vi "InitializePathsByIndex.vi"(8 "error in (no error)":errorcluster, 10 "Paths":string[](array[string]), 11 "Setting Database in":refnum<class "Setting Database.lvclass">) -> (0 "error out":errorcluster, 3 "Setting Database out":refnum<class "Setting Database.lvclass">)   [LabVIEW 2019, in "Setting Database.lvclass"]
uses:
  Setting Database.lvclass
  Setting Database.lvclass/Setting Database.ctl
  Path Settings/Path Settings.lvclass
  C:/Users/Albro/Documents/GitHub/AFM-Lithography/lvsrc/Classes/Settings/ObjectSettings/ObjectSettings.lvclass
  <vilib>/Utility/sysdir.llb/Get System Directory.vi
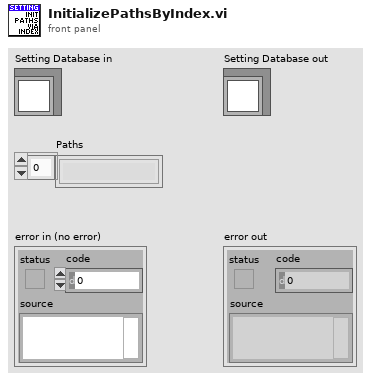
[diagram p1: front panel]
types:
  T1 = cluster{"Path":i32, "Funnel":i32, "Rectangle":i32, "Dot":i32}
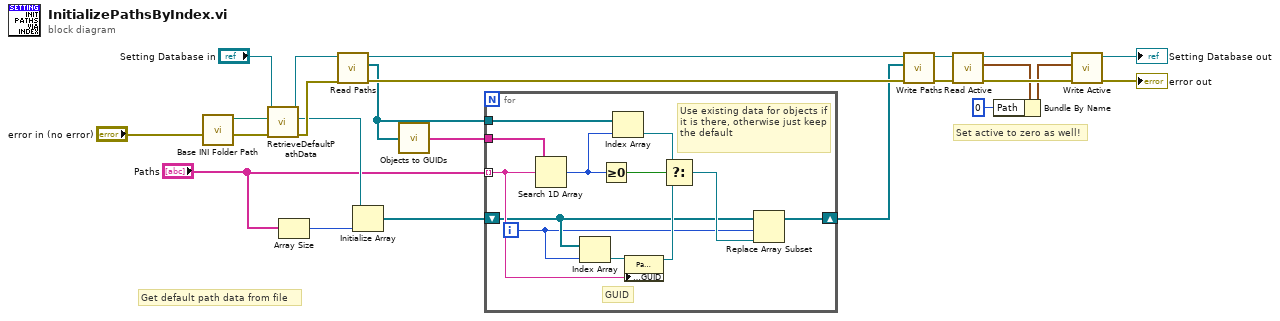
[diagram p0: block diagram]
diagram:
  # "Get default path data from file"
  # "Set active to zero as well!"
  n1 = call "Base INI Folder Path.vi"() -> ("Base Path"=w7:path)  [unwired: 11 in]
  n2 = call "RetrieveDefaultPathData.vi"("error in (no error)"="error in (no error)", "Path"=w7, "Setting Database In"="Setting Database in") -> ("error out"=w11:errorcluster, "Path Settings"=w8:refnum<class "Path Settings.lvclass">, "Setting Database Out"=w9:refnum<class "Setting Database.lvclass">)  [unwired: 6 in]
  n3 = Array Size(array="Paths") -> (size(s)=w6:i32)
  n4 = call "Read Paths.vi"("error in (no error)"=w11, "Setting Database in"=w9) -> ("error out"=w21:errorcluster, "Paths"=w5:refnum<class "Path Settings.lvclass">[], "Setting Database out"=w22:refnum<class "Setting Database.lvclass">)  [unwired: 7 in]
  n5 = Initialize Array(w8, w6) -> (w2:refnum<class "Path Settings.lvclass">[])
  n6 = call "Objects to GUIDs.vi"("Objects"=w5) -> ("GUIDs"=w4:string[])  [unwired: 3 in, 1 out]
  n7 = for {
    tunnel: w5 -> [w33]
    shift-right: [w35] -> w1
    shift-left: w2 -> [w25]
    tunnel: w4 -> [w32]
    tunnel: "Paths" -> [w30] mode=indexing
    i -> [w24]
    # "GUID"
    # "Use existing data for objects if it is there, otherwise just keep the default"
    n8 = Search 1D Array(1D array=w32, element=w30) -> (index of element=w34:i32)  [unwired: 1 in]
    n9 = Index Array(array=w25, index=w24) -> (element=w31:refnum<class "Path Settings.lvclass">)
    n10 = Greater Or Equal To 0?(x=w34) -> (x >= 0?=w29:bool)
    n11 = Index Array(array=w33, index=w34) -> (element=w28:refnum<class "Path Settings.lvclass">)
    n12 = property class="Path Settings.lvclass"(reference=w31, "Accessors:GUID"=w30) -> (reference out=w26:refnum<class "Path Settings.lvclass">)  [unwired: 1 in, 1 out]
    n13 = Select(t=w28, s=w29, f=w26) -> (s? t:f=w27:refnum<class "Path Settings.lvclass">)
    n14 = Replace Array Subset(array=w25, new element=w27, index=w24) -> (w35:refnum<class "Path Settings.lvclass">[])
  }
  n15 = call "Write Paths.vi"("error in (no error)"=w21, "Paths"=w1, "Setting Database in"=w22) -> ("error out"=w17:errorcluster, "Setting Database out"=w19:refnum<class "Setting Database.lvclass">)  [unwired: 7 in]
  n16 = call "Read Active.vi"("error in (no error)"=w17, "Setting Database in"=w19) -> ("error out"=w16:errorcluster, "Active"=w15:T1, "Setting Database out"=w18:refnum<class "Setting Database.lvclass">)  [unwired: 7 in]
  n17 = Bundle By Name(cluster=w15, "Path"=0) -> (w13:T1)
  n18 = call "Write Active.vi"("error in (no error)"=w16, "Active"=w13, "Setting Database in"=w18) -> ("error out"=→"error out":errorcluster, "Setting Database out"=→"Setting Database out":refnum<class "Setting Database.lvclass">)  [unwired: 7 in]
